vi "create overlay set.vi"(8 "error in":errorcluster, 10 "overlay glyph":string, 11 "glyph manager in":T1) -> (0 "error out":errorcluster, 3 "glyph manager out":T1)   [LabVIEW 2013, in "glyph manager.lvlib"]
uses:
  glyph manager.lvlib
  glyph manager.ctl
  <vilib>/picture/picture.llb/imagedata.ctl
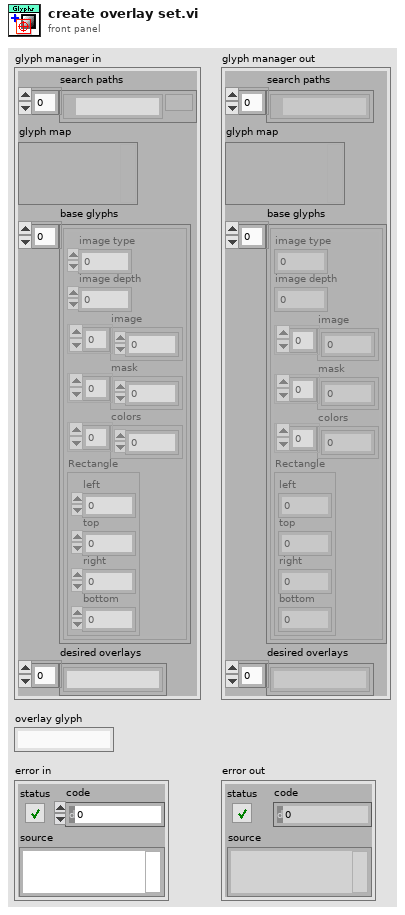
[diagram p1: front panel]
types:
  T1 = typedef "glyph manager.lvlib/glyph manager.ctl" = cluster{"search paths":path[], "glyph map":variant, "base glyphs":T2[], "desired overlays":string[]}
  T2 = typedef "imagedata.ctl" = cluster{"image type":i32, "image depth":i32, "image":u8[], "mask":u8[], "colors":u32[], "Rectangle":cluster{"left":i16, "top":i16, "right":i16, "bottom":i16}}
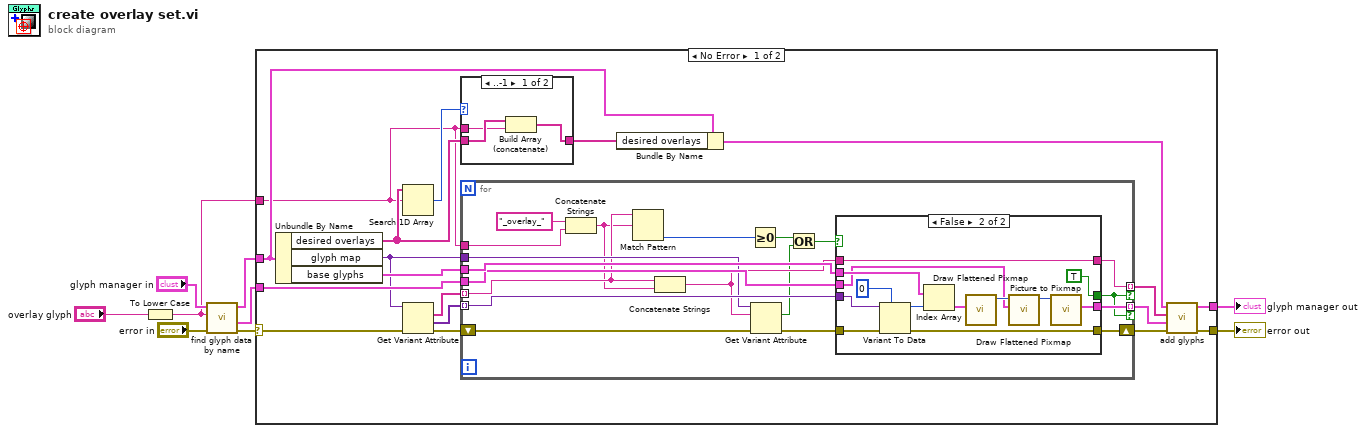
[diagram p0: block diagram]
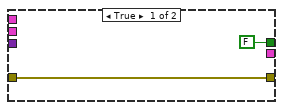
[diagram p3: hidden frame]
diagram:
  n1 = To Lower Case(string="overlay glyph") -> (all lower case string=w3:string)
  n2 = call "find glyph data by name.vi"("error in"="error in", "name"=w3, "glyph manager in"="glyph manager in") -> ("error out"=w2:errorcluster, "image data"=w1:T2, "glyph manager out"=w5:T1)  [unwired: 5 in, 1 out]
  n3 = case shown="No Error" w2 {
    selector: w2 -> [w17 w67]
    tunnel: [w22 w67] -> w7
    tunnel: [w21 w66] -> w6
    tunnel: w5 -> [w20 w66]
    tunnel: w3 -> [w12 _]
    tunnel: w1 -> [w11 _]
    frame No Error {
      n4 = Unbundle By Name(w20) -> ("desired overlays"=w14:string[], "glyph map"=w10:variant, "base glyphs"=w25:T2[])
      n5 = Search 1D Array(1D array=w14, element=w12) -> (index of element=w15:i32)  [unwired: 1 in]
      n6 = Get Variant Attribute(Variant=w10, error in=w17) -> (names=w26:string[], values=w24:variant[], error out=w27:errorcluster)  [unwired: 2 in, 1 out]
      n7 = case shown="..-1" w15 {
        tunnel: w14 -> [w30 w31]
        tunnel: [w29 w31] -> w13
        tunnel: w12 -> [w28 _]
        frame ..-1 {
          n8 = Build Array (concatenate)(w30, w28) -> (w29:string[])
        }
        frame 0.. {
        }
      }
      n9 = for {
        shift-right: [w46] -> w23
        shift-left: w27 -> [w41]
        tunnel: w26 -> [w38] mode=indexing
        tunnel: w12 -> [w43]
        tunnel: [w50] -> w19 mode=indexing if=w42
        tunnel: w25 -> [w48]
        tunnel: w24 -> [w49] mode=indexing
        tunnel: [w47] -> w18 mode=indexing if=w42
        tunnel: w11 -> [w45]
        tunnel: w10 -> [w39]
        n10 = Concatenate Strings("_overlay_" ("string"), w43) -> (w37:string)
        n11 = Match Pattern(string=w38, regular expression=w37) -> (offset past match=w34:i32)  [unwired: 1 in, 3 out]
        n12 = Concatenate Strings(w38, w37) -> (w36:string)
        n13 = Greater Or Equal To 0?(x=w34) -> (x >= 0?=w33:bool)
        n14 = Get Variant Attribute(Variant=w39, name=w36, error in=w41) -> (found=w32:bool, error out=w40:errorcluster)  [unwired: 1 in, 2 out]
        n15 = Or(x=w33, y=w32) -> (x .or. y?=w35:bool)
        n16 = case shown="False" w35 {
          tunnel: [_ w53] -> w50
          tunnel: w40 -> [w51 w65]
          tunnel: w49 -> [_ w64]
          tunnel: w48 -> [_ w62]
          tunnel: [_ w57] -> w47
          tunnel: [w51 w56] -> w46
          tunnel: w45 -> [_ w55]
          tunnel: [FALSE TRUE] -> w42
          tunnel: w36 -> [_ w53]
          frame True {
          }
          frame False {
            n17 = Variant To Data(error in=w65, type=0, Variant=w64) -> (data=w61:i32, error out=w56:errorcluster)
            n18 = Index Array(array=w62, index=w61) -> (element=w60:T2)
            n19 = call <vilib>:"Draw Flattened Pixmap.vi"("image data"=w60) -> ("new picture"=w59:picture)  [unwired: 8 in]
            n20 = call <vilib>:"Draw Flattened Pixmap.vi"("image data"=w55, "picture"=w59) -> ("new picture"=w58:picture)  [unwired: 7 in]
            n21 = call <vilib>:"Picture to Pixmap.vi"("picture"=w58) -> ("image data"=w57:T2)  [unwired: 9 in, 1 out]
          }
        }
      }
      n22 = Bundle By Name(cluster=w20, "desired overlays"=w13) -> (w16:T1)
      n23 = call "add glyphs.vi"("error in"=w23, "glyphs"=w18, "names"=w19, "glyph manager in"=w16) -> ("error out"=w22:errorcluster, "glyph manager out"=w21:T1)  [unwired: 6 in]
    }
    frame Error {
    }
  }
  "error out" <- w7
  "glyph manager out" <- w6
